vi "Is Attribute a Pointer.vi"(7 "Linked List ID":string, 8 "error in (no error)":errorcluster, 9 "Type":variant, 10 "Attribute Name":string, 11 "Linked List in":refnum<class "Linked List.lvclass">) -> (0 "error out":errorcluster, 1 "Pointer ID":string, 2 "Pointer?":bool, 3 "Linked List out":refnum<class "Linked List.lvclass">, 4 "Pointer Attribute Name":string)   [LabVIEW 2020, in "Linked Lists.lvlib" / "Linked List.lvclass"]
uses:
  <vilib>/gpm_packages/@cs/linked-list/Source/Linked List/Linked List/Linked List.lvclass
  <vilib>/gpm_packages/@cs/linked-list/Source/Linked List/Linked List Definition/Linked List Definition.lvclass
  <vilib>/gpm_packages/@cs/linked-list/Source/Linked List/Linked List/Linked List.lvclass/Linked List.ctl
  <vilib>/gpm_packages/@cs/lookup-table/Source/LookupTable/LookupTable.lvclass/LookupTable.ctl
  23411bee-76f4-42eb-bfa8-5a15a6e2d804.vi
  eac7a04f-1823-4a91-9a7b-67fc82fa7d11.vi
  <vilib>/gpm_packages/@cs/lookup-table/Source/LookupTable/Read Table Reference.vi
  23411bee-76f4-42eb-bfa8-5a15a6e2d804.vi/5a7267ad-595e-4610-9ac2-8bef780848ff.vi
  eac7a04f-1823-4a91-9a7b-67fc82fa7d11.vi/5a7267ad-595e-4610-9ac2-8bef780848ff.vi
  <vilib>/gpm_packages/@cs/lookup-table/Source/LookupTable/LookupTable.lvclass
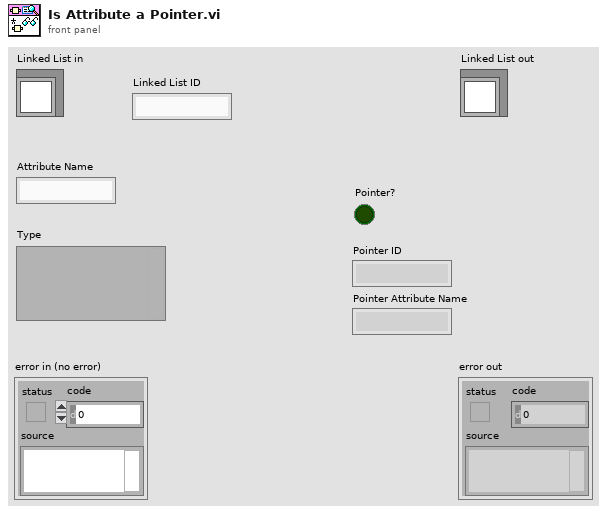
[diagram p1: front panel]
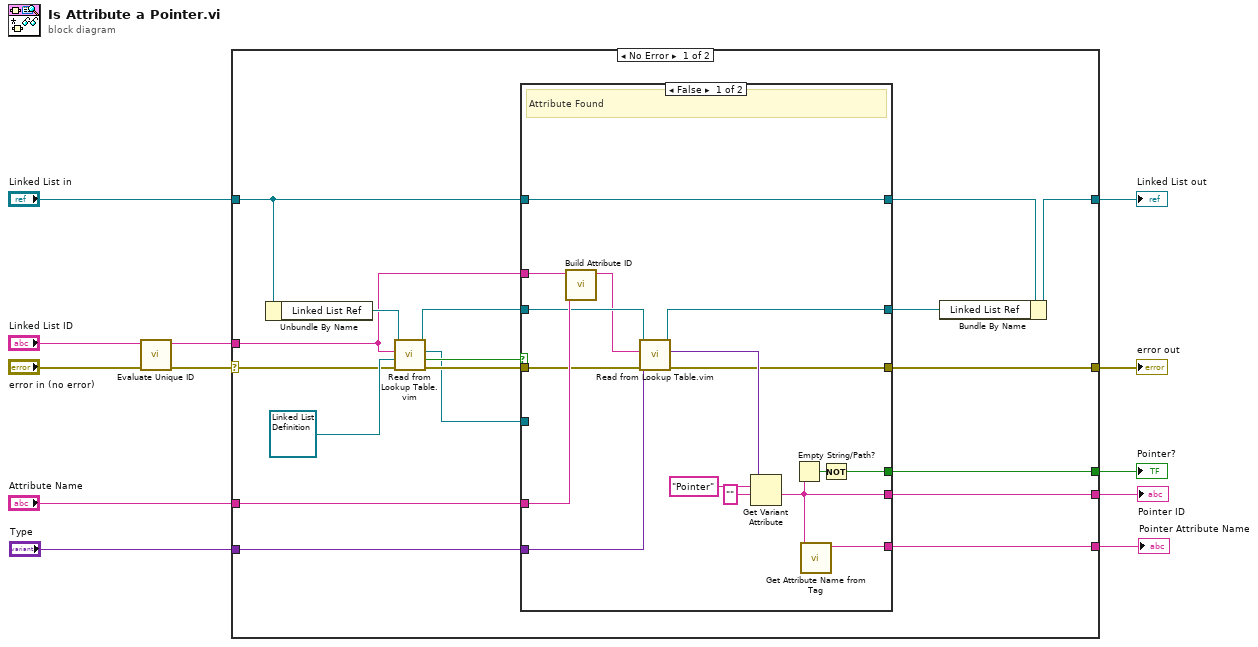
[diagram p0: block diagram]
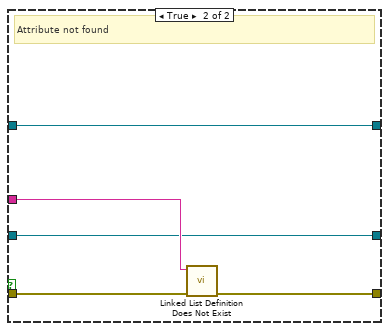
[diagram p2: hidden frame]
diagram:
  n1 = call <vilib>:"Evaluate Unique ID.vi"("error in (no error)"="error in (no error)", "Unique ID"="Linked List ID") -> ("error out"=w10:errorcluster, "Unique ID Out"=w6:string)  [unwired: 8 in]
  n2 = case shown="No Error" w10 {
    selector: w10 -> [w28 w53]
    tunnel: [w21 w53] -> w9
    tunnel: [w15 w52] -> w8
    tunnel: "Linked List in" -> [w22 w52]
    tunnel: w6 -> [w24 _]
    tunnel: "Attribute Name" -> [w20 _]
    tunnel: "Type" -> [w19 _]
    tunnel: [w18 _] -> w3
    tunnel: [w14 _] -> w2
    tunnel: [w13 _] -> w1
    frame No Error {
      n3 = Unbundle By Name(w22) -> ("Linked List Ref"=w30:refnum<data-value>)
      n4 = call "Read from Lookup Table.vim"("error in (no error)"=w28, "Type"=refnum<class "Linked List Definition.lvclass"> refnum ("Linked List.lvlib:Linked List Definition.lvclass"), "Item Name"=w24, "LookupTable Reference"=w30) -> ("error out"=w26:errorcluster, "Not Found?"=w27:bool, "Value"=w25:refnum<class "Linked List Definition.lvclass">, "LookupTable Reference Out"=w23:refnum<data-value>)  [unwired: 4 in]
      n5 = case shown="False" w27 {
        tunnel: w26 -> [w44 w51]
        tunnel: w25 -> [_ _]
        tunnel: w24 -> [w46 w49]
        tunnel: w23 -> [w43 w48]
        tunnel: w22 -> [w41 w47]
        tunnel: [w35 w50] -> w21
        tunnel: [w36 w48] -> w17
        tunnel: [w41 w47] -> w16
        tunnel: w20 -> [w45 _]
        tunnel: w19 -> [w38 _]
        tunnel: [w33 _] -> w18
        tunnel: [w32 _] -> w14
        tunnel: [w31 _] -> w13
        frame False {
          # "Attribute Found"
          n6 = call <vilib>:"Build Attribute ID.vi"("Attr Name"=w45, "Unique ID"=w46) -> ("Attr ID Out"=w42:string)  [unwired: 9 in]
          n7 = call "Read from Lookup Table.vim"("error in (no error)"=w44, "Type"=w38, "Item Name"=w42, "LookupTable Reference"=w43) -> ("error out"=w35:errorcluster, "Value"=w37:variant, "LookupTable Reference Out"=w36:refnum<data-value>)  [unwired: 4 in, 1 out]
          n8 = Get Variant Attribute(Variant=w37, name="Pointer", default value (empty Variant)="") -> (value=w32:string)  [unwired: 1 in, 3 out]
          n9 = Empty String/Path?(string/path=w32) -> (empty?=w34:bool)
          n10 = call <vilib>:"Get Attribute Name from Tag.vi"("Tag"=w32) -> ("Attribute Name"=w31:string)  [unwired: 8 in, 2 out]
          n11 = Not(x=w34) -> (.not. x?=w33:bool)
        }
        frame True {
          # "Attribute not found"
          n12 = call <vilib>:"Linked List Definition Does Not Exist.vi"("Error In"=w51, "Unique ID"=w49) -> ("Error Out"=w50:errorcluster)  [unwired: 9 in]
        }
      }
      n13 = Bundle By Name(cluster=w16, "Linked List Ref"=w17) -> (w15:refnum<class "Linked List.lvclass">)
    }
    frame Error {
    }
  }
  "error out" <- w9
  "Linked List out" <- w8
  "Pointer?" <- w3
  "Pointer ID" <- w2
  "Pointer Attribute Name" <- w1
